vi "ConfigTrigger.vi"(8 "error in (no error)":errorcluster, 11 "NiDaqMx in":refnum<class "NiDaqMx.lvclass">) -> (0 "error out":errorcluster, 3 "NiDaqMx out":refnum<class "NiDaqMx.lvclass">)   [LabVIEW 2018, in "DigitizerPlugins.lvlib" / "NiDaqMx.lvclass"]
uses:
  NiDaqMx.lvclass
  C:/projects/PMUCal/Modules/Digitizer/DigitizerPlugins/DigitizerBaseClass/DigitizerBase.lvclass
  DigitizerBaseClass/DigitizerBase.lvclass/DigitizerBase.ctl
  DigitizerBaseClass/Accessors/Read SyncInfo.vi
  DigitizerBaseClass/Accessors/Read InstRef.vi
  DigitizerBaseClass/Accessors/Read Trigger.vi
  <vilib>/Utility/error.llb/Error Cluster From Error Code.vi
  <vilib>/DAQmx/configure/trigger.llb/DAQmx Start Trigger (Digital Edge).vi
  <vilib>/DAQmx/configure/trigger.llb/DAQmx Start Trigger (None).vi
  <vilib>/DAQmx/configure/trigger.llb/DAQmx Reference Trigger (Digital Edge).vi
  <vilib>/ErrorRing/Error Ring.xnode
  <vilib>/DAQmx/configure/events/hardwareSignals.llb/DAQmx Export Signal (Most Signals).vi
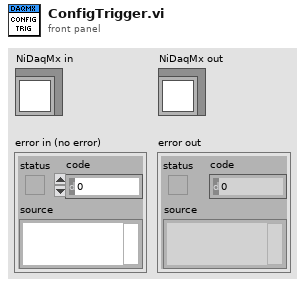
[diagram p1: front panel]
types:
  T1 = typedef "DigitizerPlugins.lvlib/DigitizerBase.lvclass/Trigger.ctl" = cluster{"Source":string, "Delay":dbl, "Holdoff":dbl, "PretriggerSamples":i32, "Sources":T2[]}
  T2 = typedef "DigitizerPlugins.lvlib/DigitizerBase.lvclass/TrigSource.ctl" = cluster{"Name":string, "Coupling":enum16{"AC", "DC", "HF Reject", "LF Reject", "Noise Reject"}, "Hysteresis":dbl, "Level":dbl, "Slope":enum16{"Positive", "Negative"}, "Type":enum16{"Edge", "Width", "Runt", "Glitch", "TV", "Window"}}
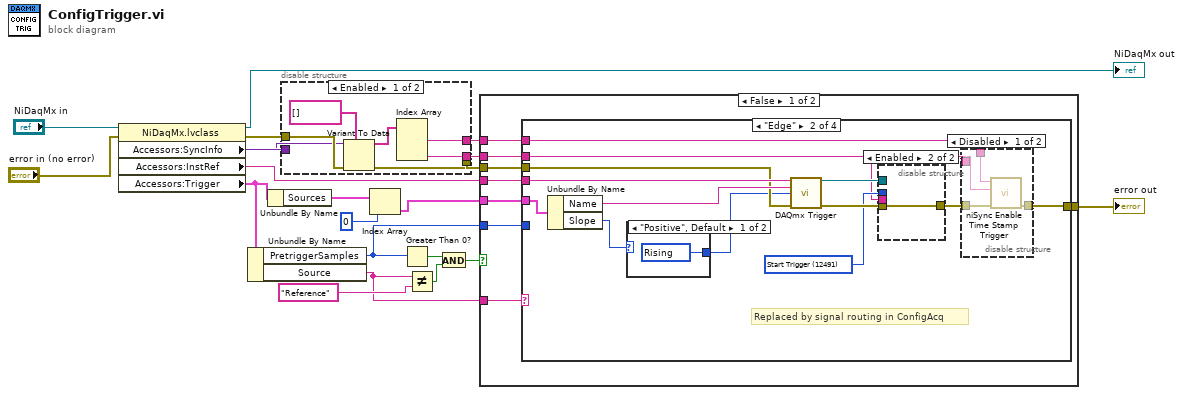
[diagram p0: block diagram]
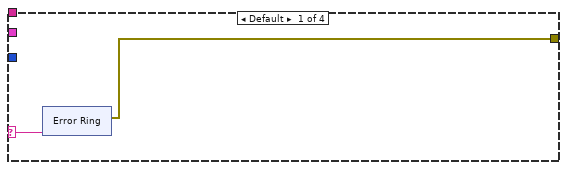
[diagram p3: hidden frame]
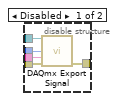
[diagram p4: hidden frame]
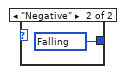
[diagram p6: hidden frame]
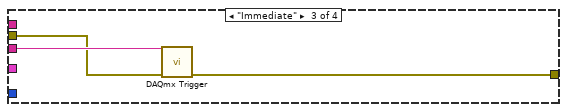
[diagram p7: hidden frame]
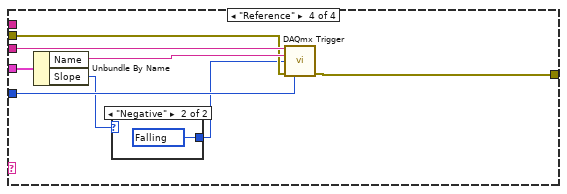
[diagram p8: hidden frame]
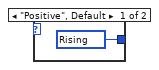
[diagram p9: hidden frame]
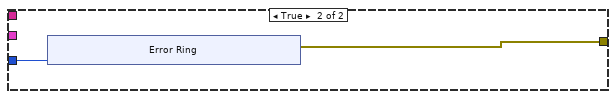
[diagram p10: hidden frame]
diagram:
  n1 = property class="NiDaqMx.lvclass"(reference="NiDaqMx in", error in="error in (no error)") -> (reference out=→"NiDaqMx out":refnum<class "NiDaqMx.lvclass">, error out=w7:errorcluster, "Accessors:SyncInfo"=w6:variant, "Accessors:InstRef"=w8:string, "Accessors:Trigger"=w10:T1)
  n2 = Unbundle By Name(w10) -> ("PretriggerSamples"=w14:i32, "Source"=w13:string)
  n3 = Unbundle By Name(w10) -> ("Sources"=w11:T2[])
  n4 = disable-structure shown="Enabled" {
    disable-tunnel: w7 -> [w27 w28]
    disable-tunnel: w6 -> [w26 _]
    disable-tunnel: [w25 w28] -> w5
    disable-tunnel: [w22 _] -> w2
    disable-tunnel: [w21 _] -> w1
    frame Enabled {
      n5 = Variant To Data(error in=w27, type=string[] [], Variant=w26) -> (data=w23:string[], error out=w25:errorcluster)
      n6 = Index Array(array=w23) -> (element #1=w21:string, element #3=w22:string)  [unwired: 3 in, 1 out]
    }
    frame Disabled {
    }
  }
  n7 = Index Array(array=w11, index=0) -> (element=w9:T2)
  n8 = Greater Than 0?(x=w14) -> (x > 0?=w18:bool)
  n9 = Not Equal?(x=w13, y="Reference") -> (x != y?=w17:bool)
  n10 = And(x=w18, y=w17) -> (x .and. y?=w15:bool)
  n11 = case shown="False" w15 {
    tunnel: w14 -> [w31 w86]
    tunnel: [w35 w85] -> w3
    tunnel: w13 -> [w36 _]
    tunnel: w9 -> [w34 _]
    tunnel: w8 -> [w33 _]
    tunnel: w5 -> [w32 _]
    tunnel: w2 -> [w30 _]
    tunnel: w1 -> [w29 _]
    frame False {
      n12 = case shown="\"Edge\"" w36 {
        selector: w36 -> [w38 _ _ _]
        tunnel: [w37 w48 w72 w80] -> w35
        tunnel: w34 -> [_ w55 _ w79]
        tunnel: w33 -> [_ w58 w74 w81]
        tunnel: w32 -> [_ w56 w73 w77]
        tunnel: w31 -> [_ _ _ w82]
        tunnel: w30 -> [_ w46 _ _]
        tunnel: w29 -> [_ w47 _ _]
        frame Default {
          n13 = xnode "Error Ring"("parameter 0"=w38) -> ("error out"=w37:errorcluster)
        }
        frame "Edge" {
          w50 = 12491 items=["AI Convert Clock"=12484, "10MHz Reference Clock"=12536, "20MHz Timebase Clock"=12486, "Sample Clock"=12487, "Advance Trigger"=12488, "Reference Trigger"=12490, "Start Trigger"=12491, "Advance Complete Event"=12492, "AI Hold Complete Event"=12493, "Counter Output Event"=12494, "Change Detection Event"=12511, "Watchdog Timer Expired Event"=12512] ("signal")
          # "Replaced by signal routing in ConfigAcq"
          n14 = Unbundle By Name(w55) -> ("Name"=w57:string, "Slope"=w54:enum16{"Positive", "Negative"})
          n15 = case shown="\"Positive\", Default" w54 {
            tunnel: [w70 w71] -> w53
            frame "Positive", Default {
              w70 = 10280 items=["Rising"=10280, "Falling"=10171] ("edge")
            }
            frame "Negative" {
              w71 = 10171 items=["Rising"=10280, "Falling"=10171] ("edge")
            }
          }
          n16 = call-poly <vilib>:"DAQmx Trigger.vi"("task/channels in"=w58, "source"=w57, "edge"=w53, "error in"=w56) -> ("task out"=w52:refnum<k21>, "error out"=w51:errorcluster)  [unwired: 10 in]
          n17 = disable-structure shown="Enabled" {
            disable-tunnel: w52 -> [w63 _]
            disable-tunnel: w51 -> [w62 w64]
            disable-tunnel: w50 -> [w61 _]
            disable-tunnel: [w60 w64] -> w49
            disable-tunnel: w46 -> [w59 _]
            frame Disabled {
              n18 = call-poly <vilib>:"DAQmx Export Signal.vi"("task/channels in"=w63, "signal"=w61, "output terminal"=w59, "error in"=w62) -> ("error out"=w60:errorcluster)  [unwired: 10 in, 1 out]
            }
            frame Enabled {
            }
          }
          n19 = disable-structure shown="Disabled" {
            disable-tunnel: w49 -> [w68 w69]
            disable-tunnel: [w67 w69] -> w48
            disable-tunnel: w47 -> [w66 _]
            disable-tunnel: w46 -> [w65 _]
            frame Disabled {
              n20 = call <instrlib>:"niSync Enable Time Stamp Trigger.vi"("error in (no error)"=w68, "terminal"=w65, "instrument handle"=w66) -> ("error out"=w67:errorcluster)  [unwired: 6 in, 1 out]
            }
            frame Enabled {
            }
          }
        }
        frame "Immediate" {
          n21 = call-poly <vilib>:"DAQmx Trigger.vi"("task/channels in"=w74, "error in"=w73) -> ("error out"=w72:errorcluster)  [unwired: 12 in, 1 out]
        }
        frame "Reference" {
          n22 = Unbundle By Name(w79) -> ("Name"=w78:string, "Slope"=w76:enum16{"Positive", "Negative"})
          n23 = case shown="\"Negative\"" w76 {
            tunnel: [w83 w84] -> w75
            frame "Positive", Default {
              w83 = 10280 items=["Rising"=10280, "Falling"=10171] ("edge")
            }
            frame "Negative" {
              w84 = 10171 items=["Rising"=10280, "Falling"=10171] ("edge")
            }
          }
          n24 = call-poly <vilib>:"DAQmx Trigger.vi"("task/channels in"=w81, "source"=w78, "edge"=w75, "error in"=w77, "pretrigger samples per channel"=w82) -> ("error out"=w80:errorcluster)  [unwired: 9 in, 1 out]
        }
      }
    }
    frame True {
      n25 = xnode "Error Ring"("parameter 0"=w86) -> ("error out"=w85:errorcluster)
    }
  }
  "error out" <- w3
